vi "Close.vi"(8 "error in (no error)":errorcluster, 11 "XNET in":refnum<class "XNET_BS120x.lvclass">) -> (0 "error out":errorcluster, 3 "XNET Out":refnum<class "XNET_BS120x.lvclass">)   [LabVIEW 2021, in "BS120x Driver.lvlib" / "XNET_BS120x.lvclass"]
uses:
  XNET_BS120x.lvclass
  XNET_BS120x.lvclass/XNET_BS120x.ctl
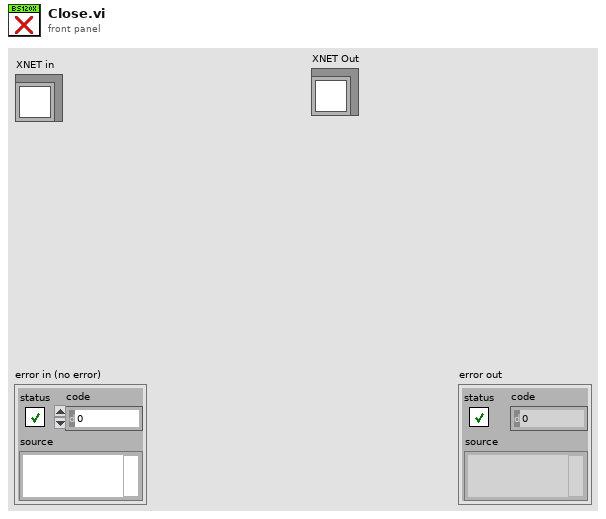
[diagram p1: front panel]
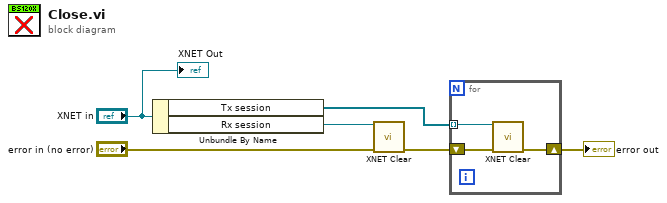
[diagram p0: block diagram]
diagram:
  n1 = Unbundle By Name("XNET in") -> ("Tx session"=w2:refnum<k21>[], "Rx session"=w5:refnum<k21>)
  n2 = call <vilib>:"XNET Clear.vi"("session in"=w5, "error in (no error)"="error in (no error)") -> ("error out"=w3:errorcluster)  [unwired: 13 in]
  n3 = for {
    tunnel: w2 -> [w8] mode=indexing
    shift-right: [w7] -> w1
    shift-left: w3 -> [w9]
    n4 = call <vilib>:"XNET Clear.vi"("session in"=w8, "error in (no error)"=w9) -> ("error out"=w7:errorcluster)  [unwired: 13 in]
  }
  "error out" <- w1
  "XNET Out" <- "XNET in"
